vi "Drive For Distance.vi"(8 "Command Iteration":i32, 9 "Speed":dbl, 10 "Distance (in)":dbl, 11 "RobotDriveDevRef":T1={"DevStatus"={"status"=FALSE, "code"=0, "source"=""}, "Motors[]"=[], "Square Inputs"=FALSE, "Max Output"=1.0}) -> (1 "Right Setpoint":dbl, 2 "Left Setpoint":dbl, 3 "Finished?":bool)   [LabVIEW 2016]
uses:
  <vilib>/Rock Robotics/WPI/RobotDrive/WPI_RobotDriveDevRef.ctl
  <vilib>/Rock Robotics/WPI/MotorControl/WPI_MotorControlDeviceRef.ctl
  <vilib>/Rock Robotics/WPI/MotorControl/WPI_MotorControlType.ctl
  <vilib>/Rock Robotics/SystemInterfaces/DIO/FPGA_DIOPWMChannel.ctl
  <vilib>/Rock Robotics/WPI/PWM/WPI_PWMDeadband.ctl
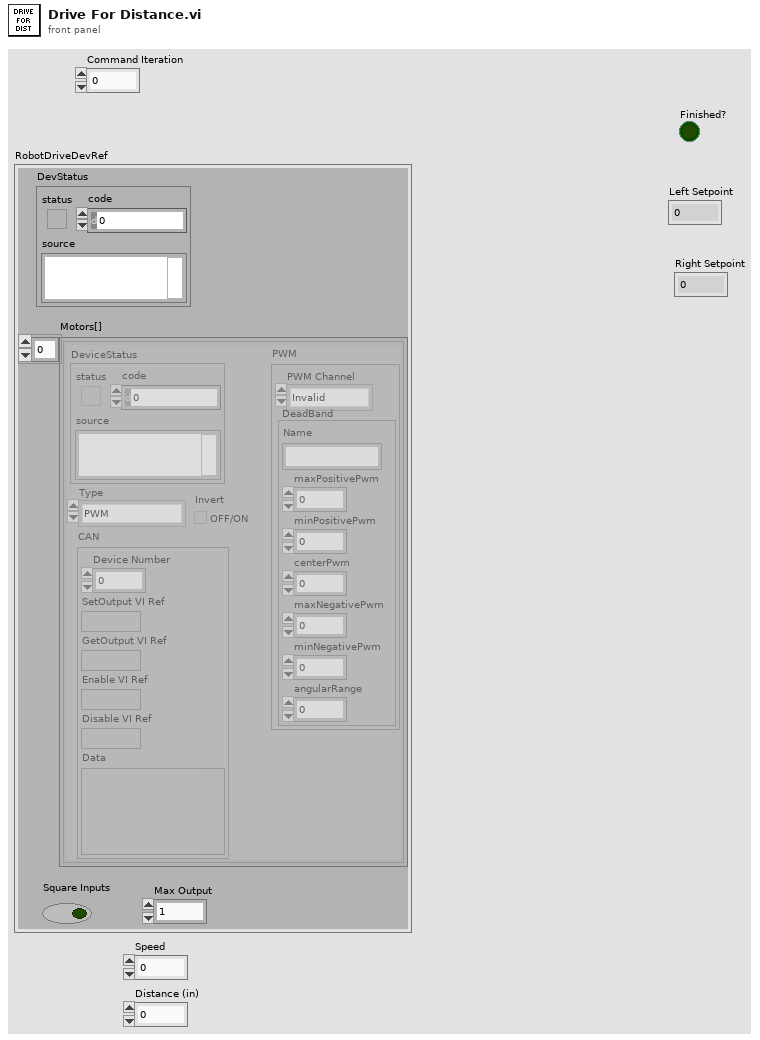
[diagram p1: front panel]
types:
  T1 = typedef "WPI_RobotDriveDevRef.ctl" = cluster{"DevStatus":errorcluster, "Motors[]":T2[], "Square Inputs":bool, "Max Output":dbl}
  T2 = typedef "WPI_MotorControlDeviceRef.ctl" = cluster{"DeviceStatus":errorcluster, "Type":T3, "PWM":cluster{"PWM Channel":T4, "DeadBand":T5}, "CAN":cluster{"Device Number":u8, "SetOutput VI Ref":variant, "GetOutput VI Ref":variant, "Enable VI Ref":variant, "Disable VI Ref":variant, "Data":variant}, "Invert":bool}
  T3 = typedef "WPI_MotorControlType.ctl" = enum16{"PWM", "CAN"}
  T4 = typedef "FPGA_DIOPWMChannel.ctl" = enum8{"PWM 0", "PWM 1", "PWM 2", "PWM 3", "PWM 4", "PWM 5", "PWM 6", "PWM 7", "PWM 8", "PWM 9", "PWM MXP 0", "PWM MXP 1", "PWM MXP 2", "PWM MXP 3", "PWM MXP 4", "PWM MXP 5", "PWM MXP 6", "PWM MXP 7", "PWM MXP 8", "PWM MXP 9", "Invalid"}
  T5 = typedef "WPI_PWMDeadband.ctl" = cluster{"Name":string, "maxPositivePwm":i32, "minPositivePwm":i32, "centerPwm":i32, "maxNegativePwm":i32, "minNegativePwm":i32, "angularRange":u16}
  T6 = typedef "WPI_CANTalonSRX_GlobalStatus.ctl" = cluster{"Applied Throttle":dbl, "Module Enabled":bool, "CAN Error":errorcluster, "Closed Loop Error":dbl, "Forward Limit Switch Closed":bool, "Reverse Limit Switch Closed":bool, "Sensor Position":dbl, "Sensor Velocity":dbl, "Current":dbl, "Sticky Fault - Over Temp":bool, "Sticky Fault - Under Voltage":bool, "Sticky Fault - Forward Limit":bool, "Sticky Fault - Reverse Limit":bool, "Sticky Fault - Forward Soft Limit":bool, "Sticky Fault - Reverse Soft Limit":bool, "Brake is Enabled":bool, "Encoder Position":dbl, "Encoder Velocity":dbl, "Encoder Index Count":dbl, "Encoder A Pin State":bool, "Encoder B Pin State":bool, "Encoder Index Pin State":bool, "Analog In":dbl, "Analog In Velocity":dbl, "Temperature (C)":dbl, "Battery Voltage":dbl, "Control 5 Is Supported":bool, "Current Profile Slot Select":dbl, "Pos Div 8":bool, "Vel Div 4":bool, "Pulse Width Position":i32, "Pulse Width Velocity":i32, "Pulse Width Rise To Rise (us)":i32, "Pulse Width Rise To Fall (us)":i32, "Mot Prof Active Is Under Run":bool, "Mot Prof Active Has Under Run":bool, "Mot Prof Active Is Last":bool, "Mot Prof Active Velocity Only":bool, "Mot Prof Active Is Valid":bool, "Mot Prof Buffer Is Full":bool, "Mot Prof Active Profile Slot Select":i32, "Mot Prof NextID":i32, "Mot Prof Count":i32, "Mot Prof Active Velocity":dbl, "Mot Prof Active Position":dbl, "Mot Prof Output Enable":i32}
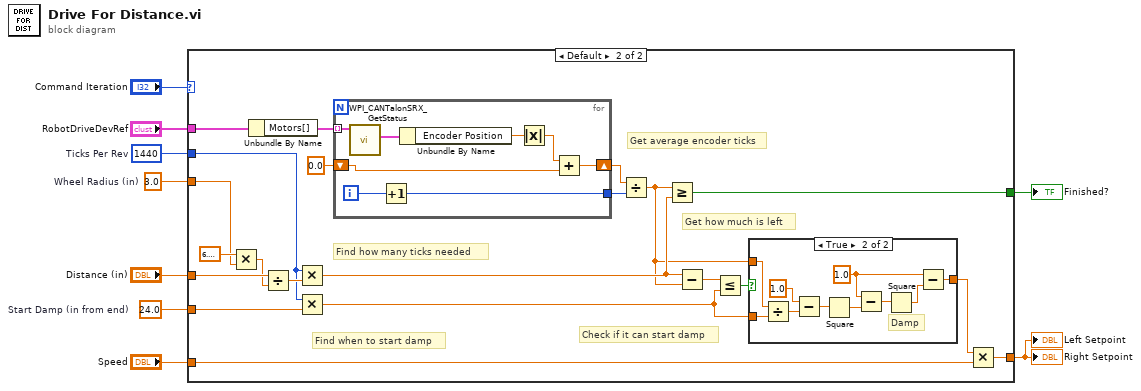
[diagram p0: block diagram]
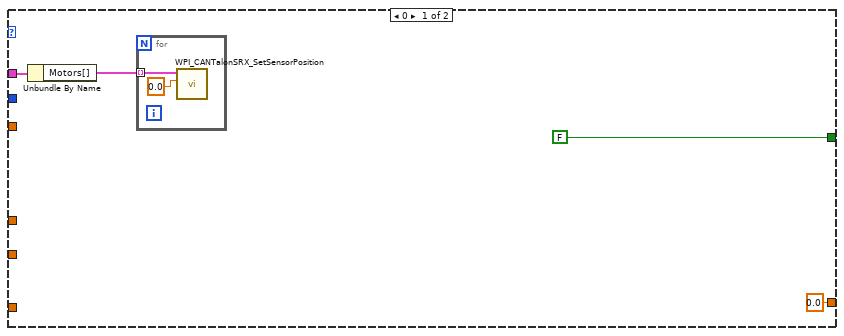
[diagram p2: hidden frame]
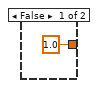
[diagram p3: hidden frame]
diagram:
  w4 = 24.0  # Start Damp (in from end)
  w7 = 3.0  # Wheel Radius (in)
  w5 = 1440  # Ticks Per Rev
  n1 = case shown="Default" "Command Iteration" {
    tunnel: "RobotDriveDevRef" -> [w13 w36]
    tunnel: w7 -> [_ w30]
    tunnel: "Distance (in)" -> [_ w29]
    tunnel: w5 -> [_ w25]
    tunnel: w4 -> [_ w26]
    tunnel: [FALSE w22] -> w2
    tunnel: "Speed" -> [_ w18]
    tunnel: [0.0 w17] -> w1
    frame 0 {
      n2 = Unbundle By Name(w13) -> ("Motors[]"=w12:T2[])
      n3 = for {
        tunnel: w12 -> [w15] mode=indexing
        n4 = call <vilib>:"WPI_CANTalonSRX_SetSensorPosition.vi"("New Sensor Position"=0.0, "CAN Talon SRX Ref"=w15) -> ()  [unwired: 8 in, 2 out]
      }
    }
    frame Default {
      # "Check if it can start damp"
      # "Get how much is left"
      # "Get average encoder ticks"
      # "Find how many ticks needed"
      # "Find when to start damp"
      n5 = Multiply(x=6.283185307179586, y=w30) -> (x*y=w28:dbl)
      n6 = Unbundle By Name(w36) -> ("Motors[]"=w35:T2[])
      n7 = Divide(x=w29, y=w28) -> (x/y=w27:dbl)
      n8 = Multiply(x=w25, y=w27) -> (x*y=w24:dbl)
      n9 = Multiply(x=w25, y=w26) -> (x*y=w20:dbl)
      n10 = for {
        tunnel: w35 -> [w53] mode=indexing
        tunnel: [w54] -> w33
        shift-right: [w52] -> w34
        shift-left: 0.0 -> [w51]
        i -> [w55]
        n11 = call <vilib>:"WPI_CANTalonSRX_GetStatus.vi"("CAN Talon SRX Ref"=w53) -> ("Talon SRX Status"=w50:T6)  [unwired: 8 in, 2 out]
        n12 = Increment(x=w55) -> (x+1=w54:i32)
        n13 = Unbundle By Name(w50) -> ("Encoder Position"=w49:dbl)
        n14 = Absolute Value(x=w49) -> (abs(x)=w48:dbl)
        n15 = Add(x=w48, y=w51) -> (x+y=w52:dbl)
      }
      n16 = Divide(x=w34, y=w33) -> (x/y=w16:dbl)
      n17 = Greater Or Equal?(x=w16, y=w24) -> (x >= y?=w22:bool)
      n18 = Subtract(x=w24, y=w16) -> (x-y=w23:dbl)
      n19 = Less Or Equal?(x=w23, y=w20) -> (x <= y?=w21:bool)
      n20 = case shown="True" w21 {
        tunnel: w16 -> [_ w43]
        tunnel: w20 -> [_ w42]
        tunnel: [1.0 w38] -> w19
        frame False {
        }
        frame True {
          w45 = 1.0
          # "Damp"
          n21 = Divide(x=w43, y=w42) -> (x/y=w41:dbl)
          n22 = Subtract(x=1.0, y=w41) -> (x-y=w39:dbl)
          n23 = Square(x=w39) -> (x^2=w47:dbl)
          n24 = Subtract(x=w45, y=w47) -> (x-y=w46:dbl)
          n25 = Square(x=w46) -> (x^2=w44:dbl)
          n26 = Subtract(x=w45, y=w44) -> (x-y=w38:dbl)
        }
      }
      n27 = Multiply(x=w19, y=w18) -> (x*y=w17:dbl)
    }
  }
  "Finished?" <- w2
  "Left Setpoint" <- w1
  "Right Setpoint" <- w1
